vi "Channel Array to Blocks.vi"(11 "Channel Descriptors":T2[](array[typedef]) {"base address" format="%016x"; "Channel Parameters"."offset" format="%d bytes"}) -> (3 "Channel Block Descriptors":T1[](array[typedef]) {"count" format="%d elements"; "First Channel Descriptor"."base address" format="%016x"; "First Channel Descriptor"."Channel Parameters"."offset" format="%d bytes"})   [LabVIEW 2017]
uses:
  Source/Shared/Typedefs/DSF.Shared.Typedefs.Configuration.Transfer.Channel Descriptor.ctl
  Source/Shared/Typedefs/DSF.Shared.Typedefs.Configuration.Transfer.Channel Parameters.ctl
  Source/Shared/Typedefs/DSF.Shared.Typedefs.Data Type.ctl
  Source/Shared/Typedefs/DSF.Shared.Typedefs.Configuration.Transfer.Channel Block Descriptor.ctl
  Source/DSF.Shared.lvlib
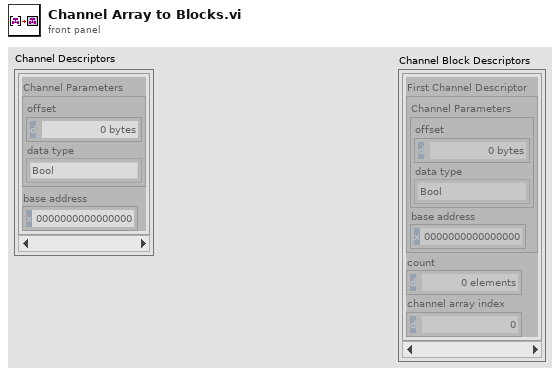
[diagram p1: front panel]
types:
  T1 = typedef "DSF.Shared.lvlib/DSF.Shared.Typedefs.Configuration.Transfer.Channel Block Descriptor.ctl" = cluster{"First Channel Descriptor":T2, "count":u64, "channel array index":u64}
  T2 = typedef "DSF.Shared.lvlib/DSF.Shared.Typedefs.Configuration.Transfer.Channel Descriptor.ctl" = cluster{"Channel Parameters":T3, "base address":u64}
  T3 = typedef "DSF.Shared.lvlib/DSF.Shared.Typedefs.Configuration.Transfer.Channel Parameters.ctl" = cluster{"offset":u64, "data type":T4}
  T4 = typedef "DSF.Shared.lvlib/DSF.Shared.Typedefs.Data Type.ctl" = enum8{"Bool", "SGL", "DBL", "I8", "I16", "I32", "I64", "U8", "U16", "U32", "U64"}
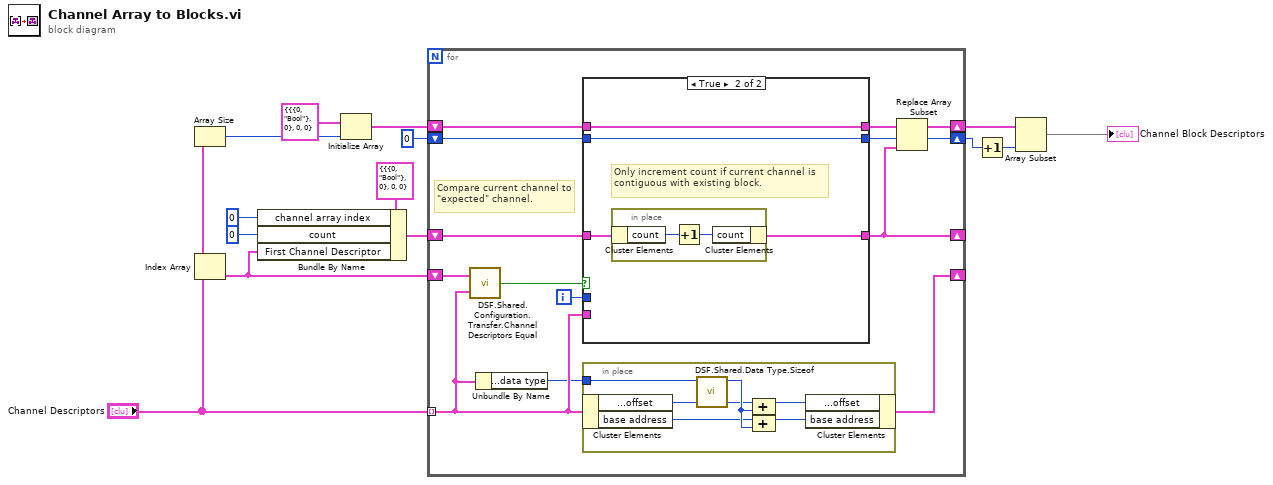
[diagram p0: block diagram]
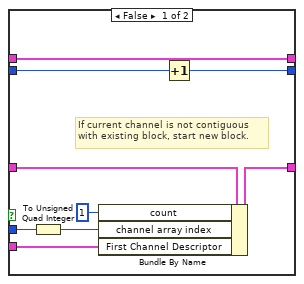
[diagram p2: hidden frame]
diagram:
  n1 = Array Size(array="Channel Descriptors") -> (size(s)=w11:i32)
  n2 = Index Array(array="Channel Descriptors") -> (element=w5:T2)  [unwired: 1 in]
  n3 = Bundle By Name(cluster=T1 {"First Channel Descriptor"={"Channel Parameters"={"offset"=0, "data type"=enum."Bool"}, "base address"=0}, "count"=0, "channel array index"=0} ("Channel Parameters"), "channel array index"=u64 0 ("index"), "count"=u64 0, "First Channel Descriptor"=w5) -> (w4:T1)
  n4 = Initialize Array(T1 {"First Channel Descriptor"={"Channel Parameters"={"offset"=0, "data type"=enum."Bool"}, "base address"=0}, "count"=0, "channel array index"=0} ("Channel Parameters"), w11) -> (w10:T1[])
  n5 = for {
    tunnel: "Channel Descriptors" -> [w17] mode=indexing
    shift-right: [w19] -> _
    shift-left: w5 -> [w18]
    shift-right: [w24] -> w8
    shift-left: w10 -> [w27]
    shift-right: [w23] -> w7
    shift-left: 0 ("size(s)") -> [w26]
    shift-right: [w22] -> _
    shift-left: w4 -> [w21]
    i -> [w20]
    # "Compare current channel to \"expected\" channel."
    n6 = call "DSF.Shared.Configuration.Transfer.Channel Descriptors Equal.vi"("Channel Descriptor 2"=w17, "Channel Descriptor 1"=w18) -> ("equal?"=w16:bool)
    n7 = Unbundle By Name(w17) -> ("Channel Parameters.data type"=w15:T4)
    n8 = case shown="True" w16 {
      tunnel: w21 -> [w40 w46]
      tunnel: [w34 w45] -> w22
      tunnel: w27 -> [w41 w44]
      tunnel: w26 -> [w42 w43]
      tunnel: [w39 w43] -> w23
      tunnel: [w41 w44] -> w25
      tunnel: w17 -> [w38 _]
      tunnel: w20 -> [w37 _]
      frame False {
        # "If current channel is not contiguous with existing block, start new block."
        n9 = To Unsigned Quad Integer(1:w37) -> (0:w35:u64)
        n10 = Bundle By Name(cluster=w40, "count"=u64 1, "channel array index"=w35, "First Channel Descriptor"=w38) -> (w34:T1)
        n11 = Increment(x=w42) -> (x+1=w39:i32)
      }
      frame True {
        # "Only increment count if current channel is contiguous with existing block."
        n12 = in-place {
          n13 = in-place-cluster #1(w46) -> ("count"=w48:u64)
          n14 = Increment(x=w48) -> (x+1=w47:u64)
          n15 = in-place-cluster #1("count"=w47) -> (w45:T1)
        }
      }
    }
    n16 = in-place {
      in-place-border: w15 -> [w29]
      n17 = in-place-cluster #2(w17) -> ("Channel Parameters.offset"=w31:u64, "base address"=w32:u64)
      n18 = call "DSF.Shared.Data Type.Sizeof.vi"("data type"=w29) -> ("size in bytes"=w33:u64)  [unwired: 9 in, 1 out]
      n19 = Compound Arithmetic op=ADD(w31, w33) -> (w28:u64)
      n20 = Compound Arithmetic op=ADD(w32, w33) -> (w30:u64)
      n21 = in-place-cluster #2("Channel Parameters.offset"=w28, "base address"=w30) -> (w19:T2)
    }
    n22 = Replace Array Subset(array=w25, new element=w22, index=w23) -> (w24:T1[])
  }
  n23 = Increment(x=w7) -> (x+1=w2:i32)
  n24 = Array Subset(array=w8, length=w2) -> (→"Channel Block Descriptors":T1[])  [unwired: 1 in]
